vi "labview_demo_error_handling.vi"(8 "error in":errorcluster, 11 "cycloneHandle":i32) -> (0 "error out":errorcluster)   [LabVIEW 2021]
uses:
  user.lib/CycloneControlSDK/CycloneControlSDK.lvlib
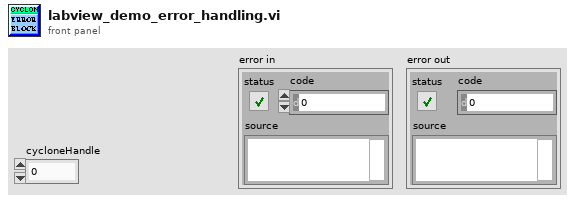
[diagram p1: front panel]
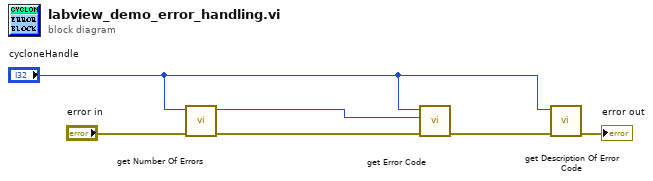
[diagram p0: block diagram]
diagram:
  n1 = call "get Number Of Errors.vi"("error in"="error in", "cycloneHandle"="cycloneHandle") -> ("error out"=w5:errorcluster, "function return"=w1:u32)  [unwired: 8 in]
  n2 = call "get Error Code.vi"("error in"=w5, "errorNum"=w1, "cycloneHandle"="cycloneHandle") -> ("error out"=w4:errorcluster)  [unwired: 7 in, 1 out]
  n3 = call "get Description Of Error Code.vi"("error in"=w4, "cycloneHandle"="cycloneHandle") -> ("error out"=→"error out":errorcluster)  [unwired: 8 in, 1 out]
